vi "RX-BPCS-SIM-UDP.vi"() -> ()   [LabVIEW 2017]
uses:
  <vilib>/Platform/TimedLoop/XDataNode/timing_clust.ctl
  <vilib>/Platform/TimedLoop/XDataNode/nitl_modes.ctl
  <vilib>/Platform/TimedLoop/XDataNode/wakeup.ctl
  <vilib>/Platform/TimedLoop/XDataNode/XDataNode.xnode
  <vilib>/Platform/TimedLoop/XDataNode/XDNodeRunTimeDep.lvlib
panel:
  in  "Stop":bool
  out "SIM-BPCS-RX-ARRAY":dbl[](array[numeric])
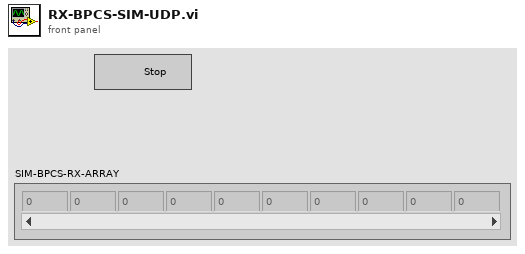
[diagram p1: front panel]
types:
  T1 = typedef "XDNodeRunTimeDep.lvlib/timing_clust.ctl" = cluster{"Expected End [f-1]":u64, "Actual End [f-1]":u64, "Finished Late? [f-1]":bool, "Expected End [i-1]":u64, "Actual End [i-1]":u64, "Finished Late? [i-1]":bool, "Expected Start [i]":u64, "Actual Start [i]":u64, "Expected Start [f]":u64, "Actual Start [f]":u64, "Source Name":string, "Structure Name":string, "Period":i64, "Deadline":i64, "Offset":i64, "Start":i64, "Priority":i32, "Timeout":i32, "Mode":T2, "Wakeup Reason":T3, "Error":errorcluster, "Source Type":string, "Secondary Source Type":string, "Global End Time":u64, "Global Start Time":u64, "Frame Duration":u64, "Iteration Duration":u64, "Assigned CPU":i32, "I/O Scan Engine Mode":u32}
  T2 = typedef "XDNodeRunTimeDep.lvlib/nitl_modes.ctl" = enum32{"No Change", "Process missed periods, maintain original phase", "Discard missed periods, maintain original phase", "Process missed periods, ignore original phase", "Discard missed periods, ignore original phase"}
  T3 = typedef "XDNodeRunTimeDep.lvlib/wakeup.ctl" = enum32{"Normal", "Aborted", "Asynchronous wakeup", "Timing source error", "Timed loop error", "Timeout"}
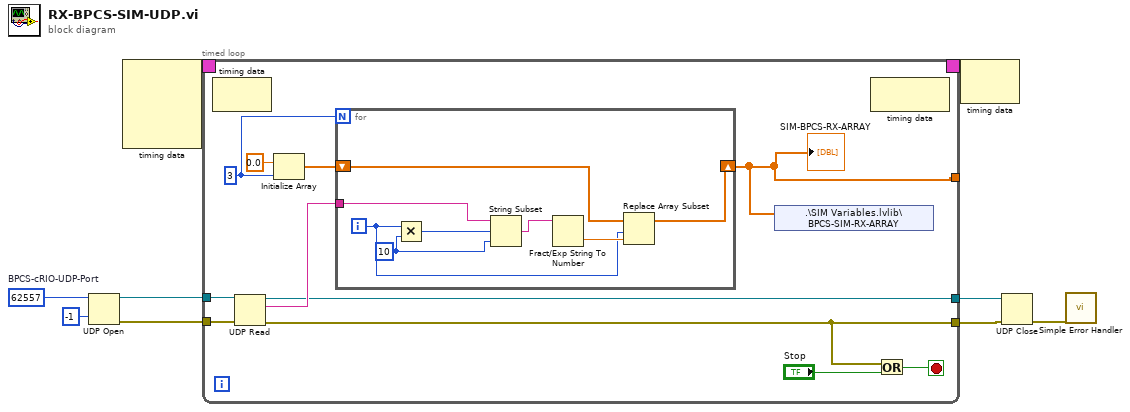
[diagram p0: block diagram]
diagram:
  w7 = u16 62557  # BPCS-cRIO-UDP-Port
  n1 = UDP Open(9:-1 ("timeout ms (25000)"), 11:w7) -> (port=w6:refnum<k16>, 0:w5:errorcluster)  [unwired: 3 in, 1 out]
  n2 = node-c288() -> (w9:T1)  [unwired: 4 in]
  n3 = timed-loop {
    timing: w9 -> [_]
    timing-out: [_] -> w8
    tunnel: w6 -> [w18]
    tunnel: w5 -> [w17]
    tunnel: [w15] -> w3
    tunnel: [w14] -> w2
    tunnel: [w10] -> _
    stop <- w19 stop-if-true
    w11 = 3 ("dimension size")
    n4 = node-c288() -> ()  [unwired: 1 in, 1 out]
    n5 = UDP Read(connection ID=w18, 8:w17) -> (data out=w16:string, error out=w14:errorcluster, 3:w15:refnum<k16>)  [unwired: 1 in, 3 out]
    n6 = Initialize Array(0.0 ("element"), w11) -> (w12:dbl[])
    n7 = for {
      N: w11 -> [_]
      tunnel: w16 -> [w27]
      shift-right: [w23] -> w10
      shift-left: w12 -> [w22]
      i -> [w24]
      w21 = 10 ("y")
      n8 = Multiply(x=w24, y=w21) -> (x*y=w26:i32)
      n9 = String Subset(string=w27, offset (0)=w26, length (rest)=w21) -> (substring=w28:string)
      n10 = Fract/Exp String To Number(string=w28) -> (number=w25:dbl)  [unwired: 3 in, 1 out]
      n11 = Replace Array Subset(array=w22, new element=w25, index=w24) -> (w23:dbl[])
    }
    "SIM-BPCS-RX-ARRAY" <- w10
    n12 = shared-variable ".\\SIM Variables.lvlib\\BPCS-SIM-RX-ARRAY"(w10) -> ()  [unwired: 1 in, 1 out]
    n13 = node-c288() -> ()  [unwired: 1 in, 1 out]
    n14 = Or(x=w14, y="Stop") -> (x .or. y?=w19:bool)
  }
  n15 = node-c288(w8) -> ()  [unwired: 1 out]
  n16 = UDP Close(connection ID=w3, 8:w2) -> (error out=w4:errorcluster)  [unwired: 1 out]
  n17 = call <vilib>:"Simple Error Handler.vi"("error in (no error)"=w4) -> ()  [unwired: 4 in, 5 out]
